vi "Day 14 - Regolith Reservoir.vi"() -> ()   [LabVIEW 2020, in "AoC 2022.lvlib"]
uses:
  AoC 2022.lvlib
panel:
  out "Sand Fall steps":T1(array[cluster])
  in  "F:Slow | T:Fast":bool=TRUE
  in  "F:Part 1 | T:Part 2":bool
  in  "Puzzle Input":string="498,4 -> 498,6 -> 496,6\n503,4 -> 502,4 -> 502,9 -> 494,9"
  out "Puzzle Part-2 Answer":string
  out "Puzzle Answer":string
  # "Press Ctrl+M & Enter the Puzzle Input and run the VI"
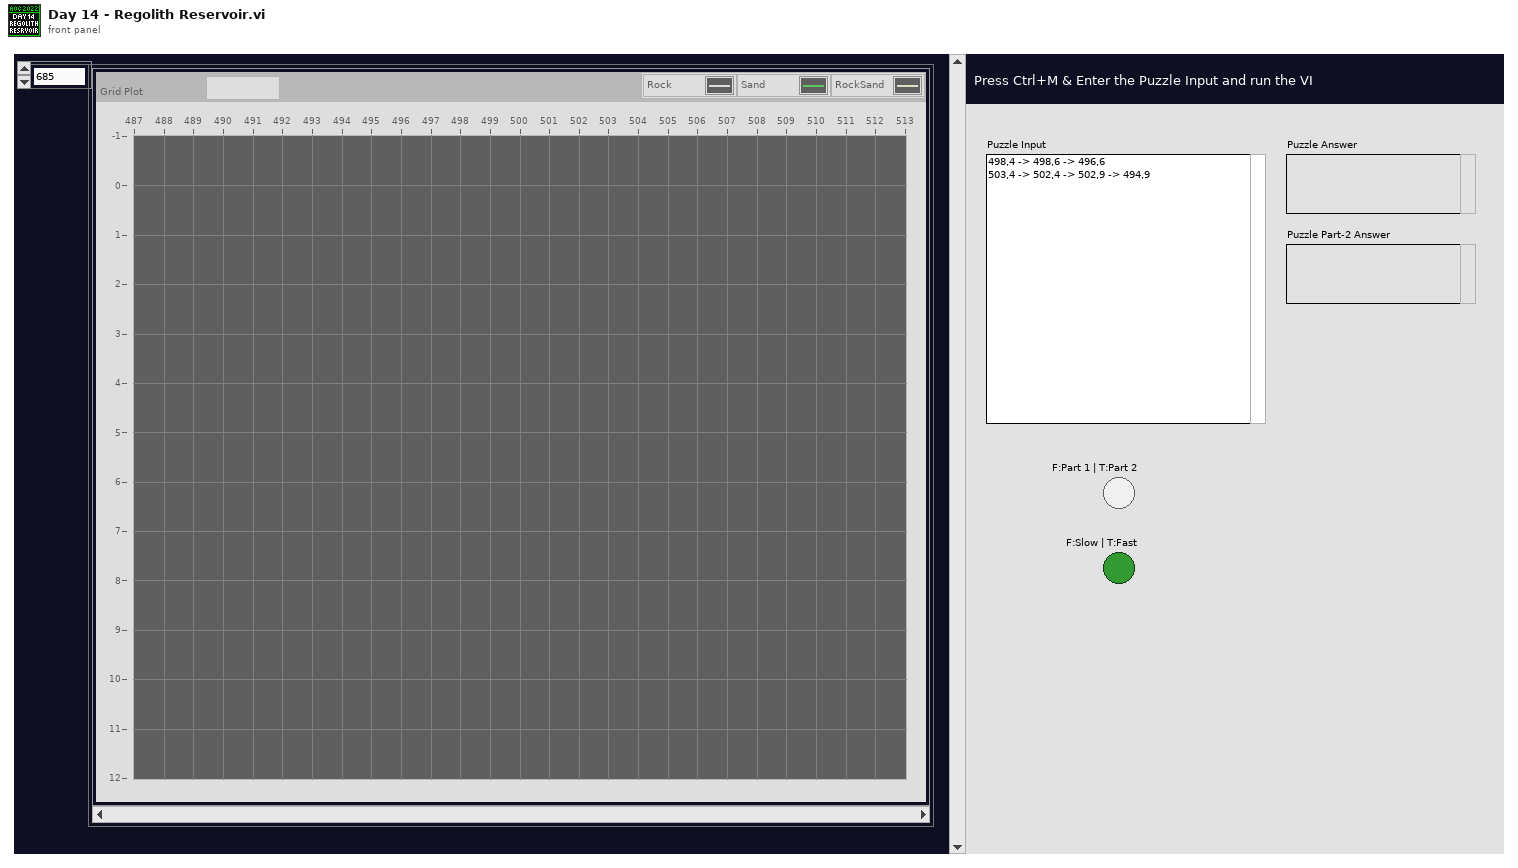
[diagram p1: front panel]
types:
  T1 = cluster{"Grid Plot":cluster{cluster{i32, i32}[]}[]}[]
  T2 = cluster{"Left":i16, "Top":i16, "Right":i16, "Bottom":i16}
  T3 = cluster{"left":i16, "top":i16, "right":i16, "bottom":i16}
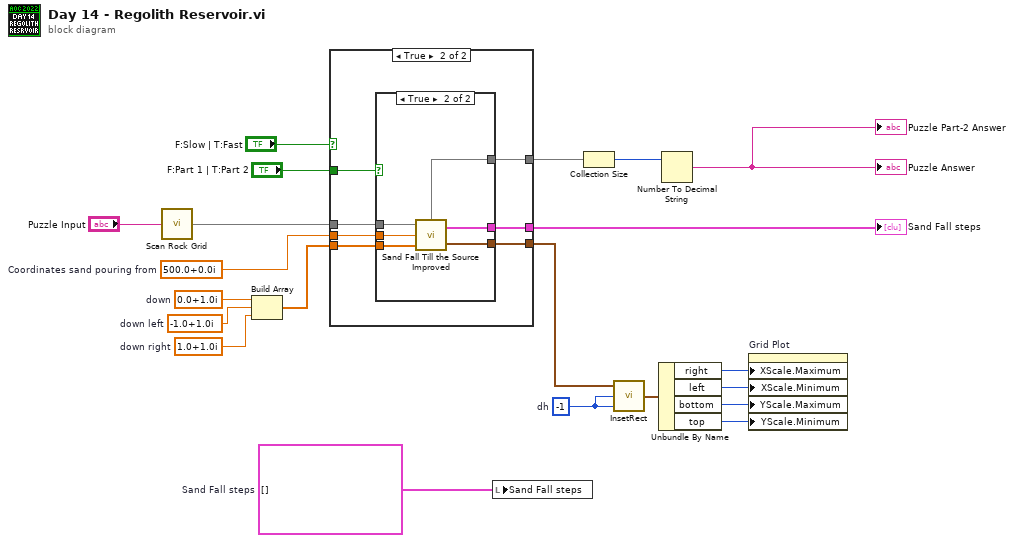
[diagram p0: block diagram]
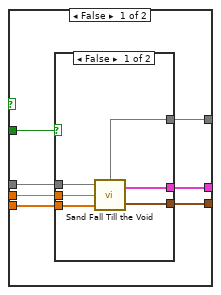
[diagram p2: hidden frame]
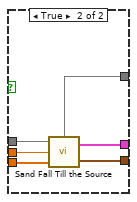
[diagram p3: hidden frame]
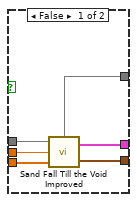
[diagram p4: hidden frame]
diagram:
  w2 = cluster{"Grid Plot":cluster{cluster[]}[]}[] []  # Sand Fall steps
  w17 = i16 -1  # dh
  w18 = cdb 1.0+1.0i  # down right
  w19 = cdb -1.0+1.0i  # down left
  w20 = cdb 0.0+1.0i  # down
  w6 = cdb 500.0+0.0i  # Coordinates sand pouring from
  n1 = call "Scan Rock Grid.vi"("Rock Scan Trace"="Puzzle Input") -> ("Rock Grid"=w7:set{cdb})
  n2 = Build Array(w20, w19, w18) -> (w5:cdb[])
  n3 = case shown="True" "F:Slow | T:Fast" {
    tunnel: [w28 w47] -> w14
    tunnel: [w27 w46] -> w9
    tunnel: [w26 w45] -> w8
    tunnel: w7 -> [w25 w44]
    tunnel: w6 -> [w24 w43]
    tunnel: w5 -> [w23 w42]
    tunnel: "F:Part 1 | T:Part 2" -> [w22 w41]
    frame False {
      n4 = case shown="False" w22 {
        tunnel: [w34 w35] -> w28
        tunnel: [w33 w36] -> w27
        tunnel: [w32 w37] -> w26
        tunnel: w25 -> [w31 w40]
        tunnel: w24 -> [w30 w38]
        tunnel: w23 -> [w29 w39]
        frame False {
          n5 = call "Sand Fall Till the Void.vi"("Possible Movements"=w29, "Sand Source Coordinates"=w30, "Rock Grid"=w31) -> ("Bounds"=w34:T2, "Sand Fall steps"=w33:cluster{"Grid Plot":cluster{cluster[]}[]}[], "Sand Grid"=w32:set{cdb})
        }
        frame True {
          n6 = call "Sand Fall Till the Source.vi"("Possible Movements"=w39, "Sand Source Coordinates"=w38, "Rock Grid"=w40) -> ("Bounds"=w35:T2, "Sand Fall steps"=w36:cluster{"Grid Plot":cluster{cluster[]}[]}[], "Sand Grid"=w37:set{cdb})
        }
      }
    }
    frame True {
      n7 = case shown="True" w41 {
        tunnel: [w53 w54] -> w47
        tunnel: [w52 w55] -> w46
        tunnel: [w51 w56] -> w45
        tunnel: w44 -> [w50 w59]
        tunnel: w43 -> [w49 w57]
        tunnel: w42 -> [w48 w58]
        frame False {
          n8 = call "Sand Fall Till the Void Improved.vi"("Possible Movements"=w48, "Sand Source Coordinates"=w49, "Rock Grid"=w50) -> ("Bounds"=w53:T2, "Sand Fall steps"=w52:cluster{"Grid Plot":cluster{cluster[]}[]}[], "Sand Grid"=w51:set{cdb})
        }
        frame True {
          n9 = call "Sand Fall Till the Source Improved.vi"("Possible Movements"=w58, "Sand Source Coordinates"=w57, "Rock Grid"=w59) -> ("Bounds"=w54:T2, "Sand Fall steps"=w55:cluster{"Grid Plot":cluster{cluster[]}[]}[], "Sand Grid"=w56:set{cdb})
        }
      }
    }
  }
  "Sand Fall steps" <- w9
  n10 = local write "Sand Fall steps"(w2) -> ()
  n11 = Collection Size(1:w8) -> (0:w15:i32)
  n12 = call <vilib>:"InsetRect.vi"("dv"=w17, "dh"=w17, "rect"=w14) -> ("inset rect"=w16:T3)
  n13 = Unbundle By Name(w16) -> ("right"=w13:i16, "left"=w12:i16, "bottom"=w11:i16, "top"=w10:i16)
  n14 = Number To Decimal String(number=w15) -> (decimal integer string=→"Puzzle Answer" →"Puzzle Part-2 Answer":string)  [unwired: 1 in]
  n15 = property on="Grid Plot" class="XYGraph (strict)"("XScale.Maximum"=w13, "XScale.Minimum"=w12, "YScale.Maximum"=w11, "YScale.Minimum"=w10) -> ()  [unwired: 2 in, 2 out]
